vi "FRCts20_EspEngine_Request.vi"(8 "error in (no error)":errorcluster, 10 "Request":T1, 11 "httpRequestID":u32) -> (0 "error out":errorcluster, 3 "httpRequestID":u32)   [LabVIEW 2014, in "FRCts20_EspEngine.lvlib"]
uses:
  FRCts20_EspEngine.lvlib
  TypeDefs/FRCts20_EspEngine_Request.ctl
  Web Methods/source/VI Source/Web Method Public Interface/FRCts20_WebMethods_ctl_request.ctl
  Backend/source/VI Source/FRCts20_Backend_API/FRCts20_Backend_API_Status.ctl
  <vilib>/wsapi/subVIs/Set Integer ESP Variable.vi
  <vilib>/wsapi/subVIs/Set String ESP Variable.vi
  FRCts20_EspEngine_FormatArrayOfKeysStrings.vi
  FRCts20_EspEngine_FormatArrayOfKeysInts.vi
  <vilib>/wsapi/NI_WebServices.lvlib
  Backend/source/VI Source/FRCts20_Backend_API/FRCts20_Backend_API.lvlib
  Web Methods/source/VI Source/FRCts20_WebMethods.lvlib
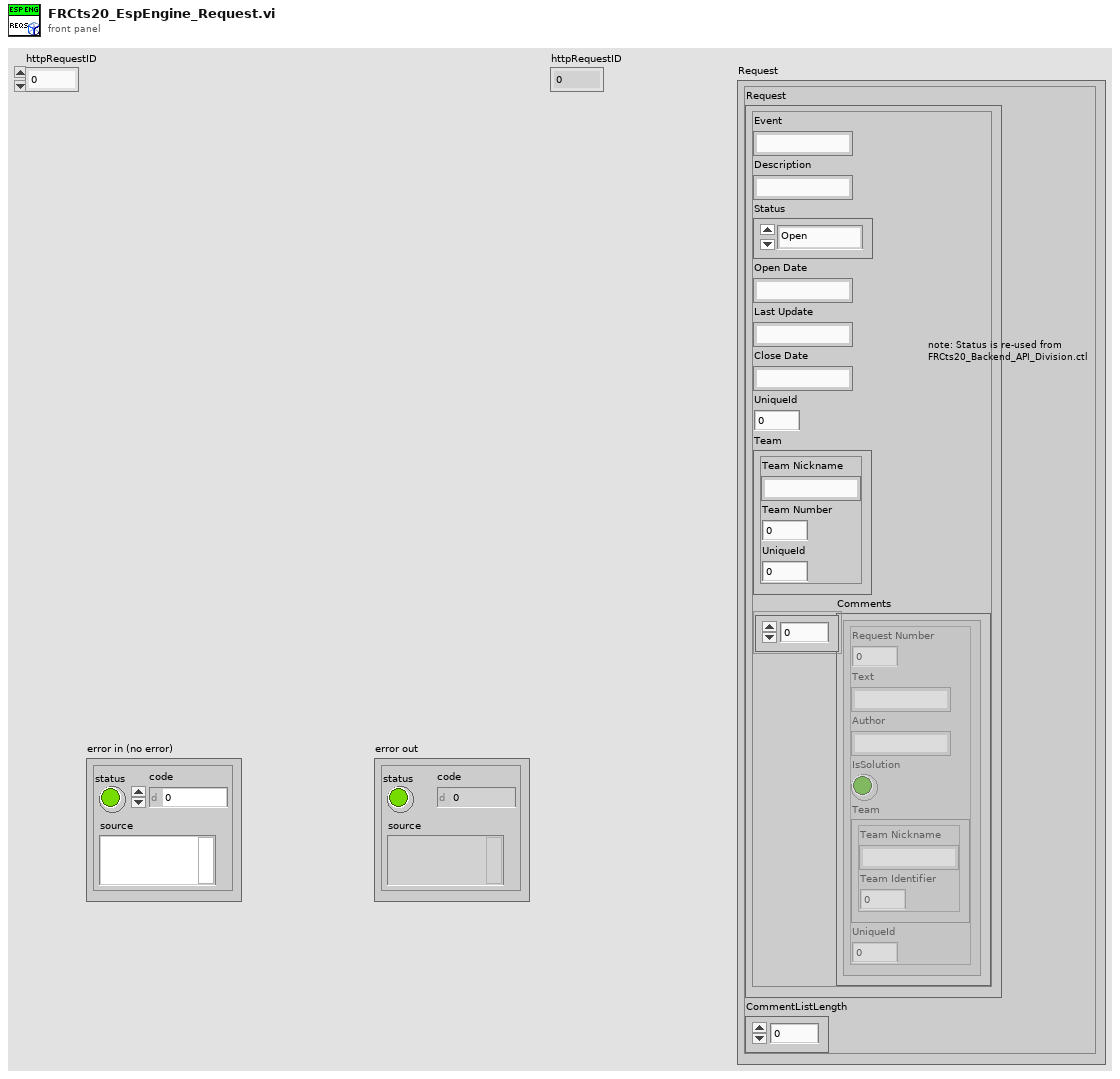
[diagram p1: front panel]
types:
  T1 = typedef "FRCts20_EspEngine.lvlib/FRCts20_EspEngine_Request.ctl" = cluster{"Request":T2, "CommentListLength":i16}
  T2 = typedef "FRCts20_WebMethods.lvlib/FRCts20_WebMethods_ctl_request.ctl" = cluster{"Event":string, "Description":string, "Status":T3, "Open Date":string, "Last Update":string, "Close Date":string, "UniqueId":i32, "Team":cluster{"Team Nickname":string, "Team Number ":i32, "UniqueId":i32}, "Comments":cluster{"Request Number":dbl, "Text":string, "Author":string, "IsSolution":bool, "Team":cluster{"Team Nickname":string, "Team Identifier ":dbl}, "UniqueId":i32}[]}
  T3 = typedef "FRCts20_Backend_API.lvlib/FRCts20_Backend_API_Status.ctl" = enum16{"Open", "In Work", "Closed"}
  T4 = cluster{"Team Nickname":string, "Team Number ":i32, "UniqueId":i32}
  T5 = cluster{"Request Number":dbl, "Text":string, "Author":string, "IsSolution":bool, "Team":cluster{"Team Nickname":string, "Team Identifier ":dbl}, "UniqueId":i32}[]
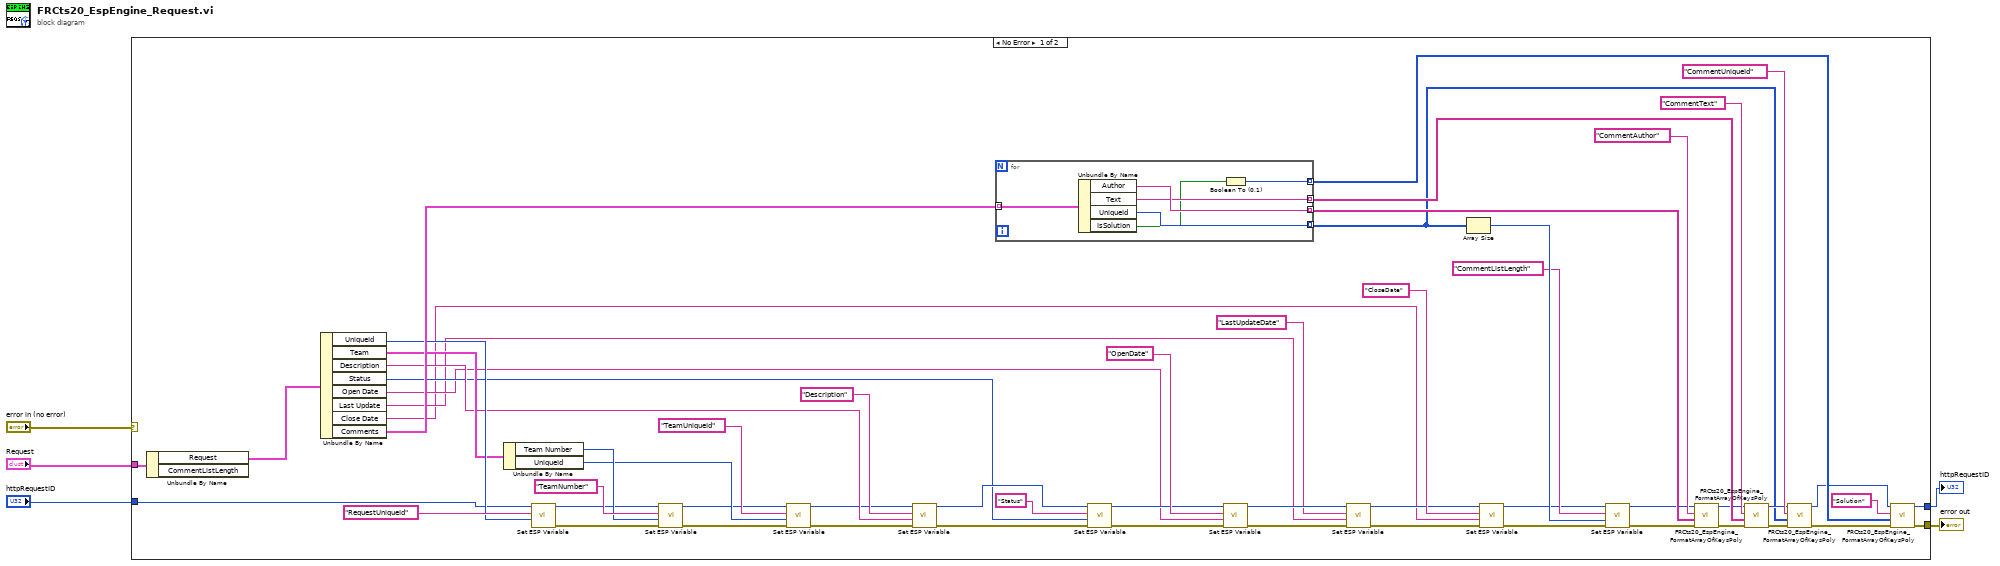
[diagram p0: block diagram]
diagram:
  n1 = case shown="No Error" "error in (no error)" {
    selector: "error in (no error)" -> [_ w69]
    tunnel: [w14 w69] -> w5
    tunnel: "Request" -> [w62 _]
    tunnel: [w15 _] -> w1
    tunnel: "httpRequestID" -> [w13 _]
    frame No Error {
      n2 = Unbundle By Name(w62) -> ("Request"=w61:T2)  [unwired: 1 out]
      n3 = Unbundle By Name(w61) -> ("UniqueId"=w58:i32, "Team"=w57:T4, "Description"=w47:string, "Status"=w41:T3, "Open Date"=w37:string, "Last Update"=w33:string, "Close Date"=w29:string, "Comments"=w60:T5)
      n4 = Unbundle By Name(w57) -> ("Team Number"=w52:i32, "UniqueId"=w51:i32)
      n5 = call-poly <vilib>:"Set ESP Variable.vi"("value"=w58, "key"="RequestUniqueId", "httpRequestID"=w13) -> ("error out"=w56:errorcluster, "httpRequestID out"=w49:u32)  [unwired: 7 in]
      n6 = call-poly <vilib>:"Set ESP Variable.vi"("error in (no error)"=w56, "value"=w52, "key"="TeamNumber", "httpRequestID"=w49) -> ("error out"=w55:errorcluster, "httpRequestID out"=w50:u32)  [unwired: 6 in]
      n7 = call-poly <vilib>:"Set ESP Variable.vi"("error in (no error)"=w55, "value"=w51, "key"="TeamUniqueId", "httpRequestID"=w50) -> ("error out"=w45:errorcluster, "httpRequestID out"=w46:u32)  [unwired: 6 in]
      n8 = call-poly <vilib>:"Set ESP Variable.vi"("error in (no error)"=w45, "value"=w47, "key"="Description", "httpRequestID"=w46) -> ("error out"=w44:errorcluster, "httpRequestID out"=w42:u32)  [unwired: 6 in]
      n9 = for {
        tunnel: w60 -> [w68] mode=indexing
        tunnel: [w67] -> w27 mode=indexing
        tunnel: [w66] -> w22 mode=indexing
        tunnel: [w65] -> w12 mode=indexing
        tunnel: [w63] -> w20 mode=indexing
        n10 = Unbundle By Name(w68) -> ("Author"=w67:string, "Text"=w66:string, "UniqueId"=w65:i32, "IsSolution"=w64:bool)
        n11 = Boolean To (0,1)(Boolean=w64) -> (0, 1=w63:i16)
      }
      n12 = call-poly <vilib>:"Set ESP Variable.vi"("error in (no error)"=w44, "value"=w41, "key"="Status", "httpRequestID"=w42) -> ("error out"=w38:errorcluster, "httpRequestID out"=w39:u32)  [unwired: 6 in]
      n13 = call-poly <vilib>:"Set ESP Variable.vi"("error in (no error)"=w38, "value"=w37, "key"="OpenDate", "httpRequestID"=w39) -> ("error out"=w36:errorcluster, "httpRequestID out"=w35:u32)  [unwired: 6 in]
      n14 = call-poly <vilib>:"Set ESP Variable.vi"("error in (no error)"=w36, "value"=w33, "key"="LastUpdateDate", "httpRequestID"=w35) -> ("error out"=w32:errorcluster, "httpRequestID out"=w30:u32)  [unwired: 6 in]
      n15 = Array Size(array=w12) -> (size(s)=w11:i32)
      n16 = call-poly <vilib>:"Set ESP Variable.vi"("error in (no error)"=w32, "value"=w29, "key"="CloseDate", "httpRequestID"=w30) -> ("error out"=w9:errorcluster, "httpRequestID out"=w8:u32)  [unwired: 6 in]
      n17 = call-poly <vilib>:"Set ESP Variable.vi"("error in (no error)"=w9, "value"=w11, "key"="CommentListLength", "httpRequestID"=w8) -> ("error out"=w6:errorcluster, "httpRequestID out"=w7:u32)  [unwired: 6 in]
      n18 = call-poly "FRCts20_EspEngine_FormatArrayOfKeysPoly.vi"("error IO"=w6, "Values"=w27, "KeyBaseName"="CommentAuthor", "httpRequestID"=w7) -> ("error IO"=w26:errorcluster, "httpRequestID out"=w18:u32)  [unwired: 6 in]
      n19 = call-poly "FRCts20_EspEngine_FormatArrayOfKeysPoly.vi"("error IO"=w26, "Values"=w22, "KeyBaseName"="CommentText", "httpRequestID"=w18) -> ("error IO"=w25:errorcluster, "httpRequestID out"=w17:u32)  [unwired: 6 in]
      n20 = call-poly "FRCts20_EspEngine_FormatArrayOfKeysPoly.vi"("error IO"=w25, "Values"=w12, "KeyBaseName"="CommentUniqueId", "httpRequestID"=w17) -> ("error IO"=w24:errorcluster, "httpRequestID out"=w16:u32)  [unwired: 6 in]
      n21 = call-poly "FRCts20_EspEngine_FormatArrayOfKeysPoly.vi"("error IO"=w24, "Values"=w20, "KeyBaseName"="Solution", "httpRequestID"=w16) -> ("error IO"=w14:errorcluster, "httpRequestID out"=w15:u32)  [unwired: 6 in]
    }
    frame Error {
    }
  }
  "error out" <- w5
  "httpRequestID" <- w1
